vi "libssh2_agent_list_identities.vi"(8 "error in (no error)":errorcluster, 11 "agent":T1) -> (0 "error out":errorcluster)   [LabVIEW 2013, in "libssh2.lvlib"]
doc: "Requests the list of public keys from an ssh agent and stores them in an internal collection."
uses:
  libssh2.lvlib
  Agent Refnum.ctl
  Not An Agent.vi
  <vilib>/Utility/error.llb/Error Cluster From Error Code.vi
  Global Settings.vi
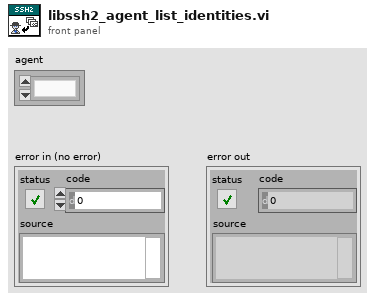
[diagram p1: front panel]
types:
  T1 = typedef "libssh2.lvlib/Agent Refnum.ctl" = refnum<k1>
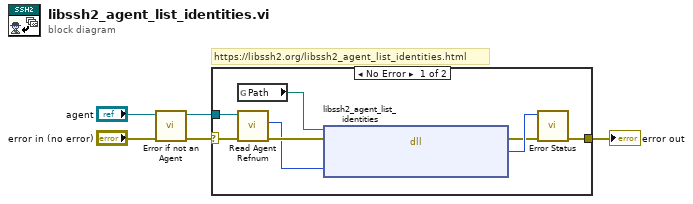
[diagram p0: block diagram]
diagram:
  # "https://libssh2.org/libssh2_agent_list_identities.html"
  n1 = call "Error if not an Agent.vi"("error in (no error)"="error in (no error)", "agent"="agent") -> ("error out"=w3:errorcluster, "agent out"=w2:T1)  [unwired: 8 in]
  n2 = case shown="No Error" w3 {
    selector: w3 -> [w12 w14]
    tunnel: [w13 w14] -> w5
    tunnel: w2 -> [w11 _]
    frame No Error {
      n3 = global read "Global Settings.vi" "Path"() -> (w8:path)
      n4 = call "Read Agent Refnum.vi"("error in (no error)"=w12, "agent"=w11) -> ("error out"=w7:errorcluster, "LIBSSH2_AGENT*"=w6:u64)  [unwired: 8 in]
      n5 = dll-call lib="?" fn="libssh2_agent_list_identities"(path in=w8, error in=w7, "agent"=w6) -> (error out=w9:errorcluster, "return value"=w10:i32)  [unwired: 2 in, 1 out]
      n6 = call "Error Status.vi"("error in (no error)"=w9, "return value"=w10) -> ("error out"=w13:errorcluster)  [unwired: 8 in, 1 out]
    }
    frame Error {
    }
  }
  "error out" <- w5
